vi "Set Group Jerk.vi"(4 "error in (no error)":errorcluster, 5 "Vector Jerk (0 units/s^3)":dbl min=0.0 max=2000000000.0 format="%.4g", 6 "Group Number (1)":i32=1 min=1, 7 "VISA resource name":refnum<visa-resource-name>) -> (0 "error out":errorcluster, 3 "VISA resource name out":refnum<visa-resource-name>)   [LabVIEW 2010, in "Newport ESP301.lvlib"]
doc: "This command is used to set the vectorial jerk value for a group. This value will be used during coordinated motion of axes assigned to the group. It will override any original jerk values specified for individual axes using JK command. The axes’ original values will be restored when the group to which they have been assigned is deleted.\nIf vectorial jerk is set to zero, a trapezoid velocity profile is employed during motion. Otherwise, an S-curve velocity profile is employed.\nThis command takes effect immediately. It can be executed when controller is idling or motion is in progress or inside a program.\n<B>Note:</B> Avoid changing jerk during acceleration or deceleration phases of a move. For better predictable results, change jerk only when all the axes assigned to this group are not in motion."
uses:
  <userlib>/Newport ESP301/Newport ESP301.lvlib
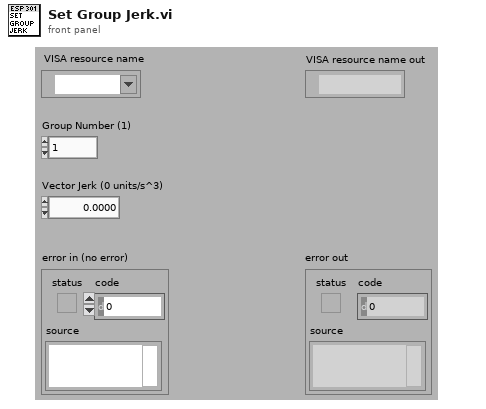
[diagram p1: front panel]
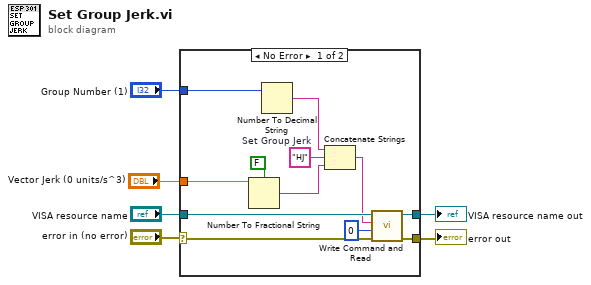
[diagram p0: block diagram]
diagram:
  n1 = case shown="No Error" "error in (no error)" {
    selector: "error in (no error)" -> [w15 w20]
    tunnel: [w17 w20] -> w6
    tunnel: "VISA resource name" -> [w18 w19]
    tunnel: [w16 w19] -> w5
    tunnel: "Group Number (1)" -> [w11 _]
    tunnel: "Vector Jerk (0 units/s^3)" -> [w8 _]
    frame No Error {
      w14 = "HJ"  # Set Group Jerk
      n2 = Number To Fractional String(use system decimal point (T)=FALSE ("utiliser le séparateur décimal du système (V)"), number=w8) -> (F-format string=w9:string)  [unwired: 2 out]
      n3 = Number To Decimal String(number=w11) -> (decimal integer string=w13:string)  [unwired: 1 in]
      n4 = Concatenate Strings(w13, w14, w9) -> (w12:string)
      n5 = call <userlib>:"Write Command and Read.vi"("error in (no error)"=w15, "Bytes to read (100)"=u32 0, "Command"=w12, "VISA resource name"=w18) -> ("error out"=w17:errorcluster, "VISA resource name out"=w16:refnum<visa-resource-name>)  [unwired: 3 in, 1 out]
    }
    frame Error {
    }
  }
  "error out" <- w6
  "VISA resource name out" <- w5
